vi "SafeBounds.vi"(5 "System no.":i32=1 min=1 step=1, 6 "Position":dbl[](array[numeric]), 7 "Type of movement":enum16{"Relative -", "Relative +", "Absolute"}(ring), 8 "Axes to move":string[](array[string]), 9 "Move":dbl[](array[numeric]), 10 "SafeMax":dbl[](array[numeric]) format="%.6f", 11 "SafeMin":dbl[](array[numeric]) format="%.6f") -> (1 "Faulty Axes":string, 2 "Message":string, 3 "All good?":bool)   [LabVIEW 2013]
panel:
  out "Moveable Axes":string[](array[string])
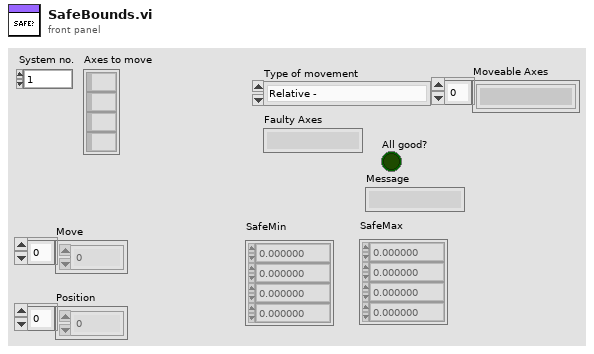
[diagram p1: front panel]
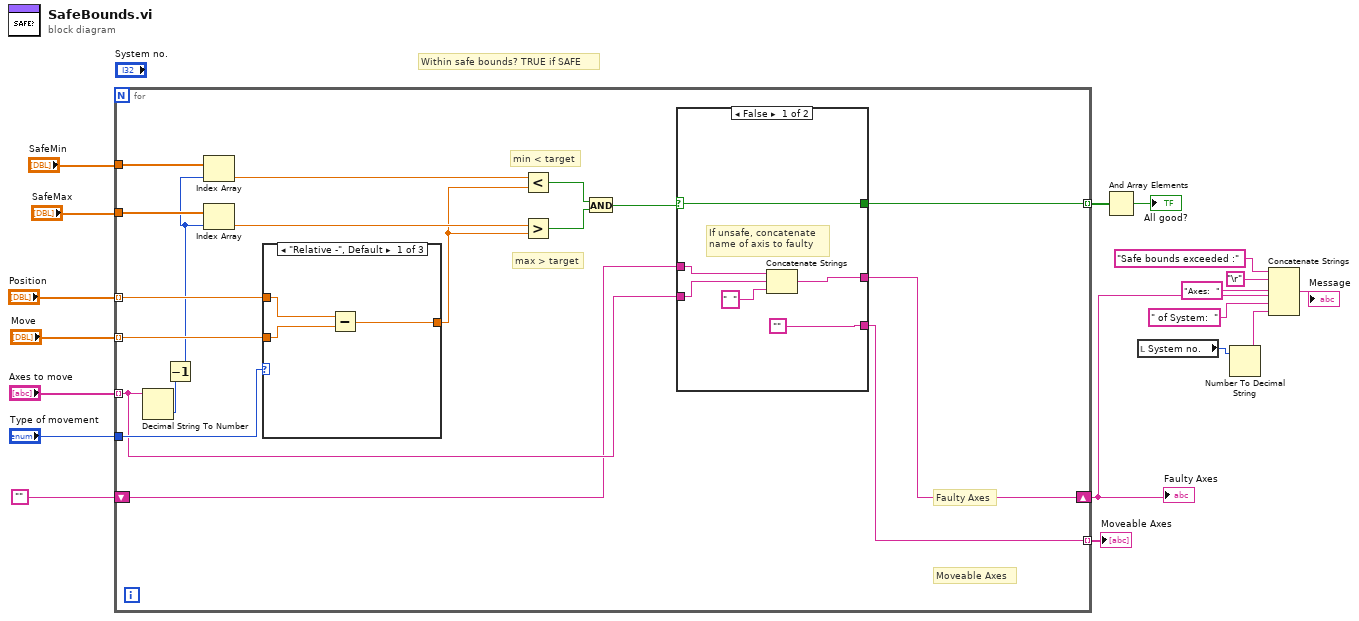
[diagram p0: block diagram]
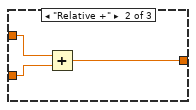
[diagram p3: hidden frame]
diagram:
  # "Within safe bounds? TRUE if SAFE"
  n1 = for {
    tunnel: "Axes to move" -> [w26] mode=indexing
    tunnel: "Position" -> [w21] mode=indexing
    tunnel: "Move" -> [w22] mode=indexing
    tunnel: "SafeMin" -> [w36]
    tunnel: "SafeMax" -> [w35]
    tunnel: "Type of movement" -> [w28]
    shift-right: [w24] -> w8
    shift-left: "" -> [w25]
    tunnel: [w23] -> w11 mode=indexing
    tunnel: [w19] -> w1 mode=indexing
    # "Moveable Axes"
    # "Faulty Axes"
    # "max > target"
    # "min < target"
    n2 = Decimal String To Number(string=w26) -> (number=w34:i32)  [unwired: 2 in, 1 out]
    n3 = Decrement(x=w34) -> (x-1=w20:i32)
    n4 = Index Array(array=w36, index=w20) -> (element=w32:dbl)
    n5 = Index Array(array=w35, index=w20) -> (element=w33:dbl)
    n6 = case shown="\"Relative -\", Default" w28 {
      tunnel: w21 -> [w48 w51 _]
      tunnel: [w47 w50 w52] -> w31
      tunnel: w22 -> [w46 w49 w52]
      frame "Relative -", Default {
        n7 = Subtract(x=w48, y=w46) -> (x-y=w47:dbl)
      }
      frame "Relative +" {
        n8 = Add(x=w51, y=w49) -> (x+y=w50:dbl)
      }
      frame "Absolute" {
      }
    }
    n9 = Less?(x=w32, y=w31) -> (x < y?=w30:bool)
    n10 = Greater?(x=w33, y=w31) -> (0:w29:bool)
    n11 = And(x=w30, y=w29) -> (x .and. y?=w27:bool)
    n12 = case shown="False" w27 {
      selector: w27 -> [w40 w44]
      tunnel: w26 -> [w38 w43]
      tunnel: w25 -> [w42 w45]
      tunnel: [w41 w45] -> w24
      tunnel: [w40 w44] -> w23
      tunnel: ["" w43] -> w19
      frame False {
        # "If unsafe, concatenate \nname of axis to faulty"
        n13 = Concatenate Strings(w42, w38, "  " ("string")) -> (w41:string)
      }
      frame True {
        # "If safe, don't concatenate \nname of axis to faulty"
      }
    }
  }
  "Faulty Axes" <- w8
  "Moveable Axes" <- w1
  n14 = And Array Elements(Boolean array=w11) -> (logical AND=→"All good?":bool)
  n15 = local read "System no."() -> (w6:i32)
  n16 = Number To Decimal String(number=w6) -> (decimal integer string=w5:string)  [unwired: 1 in]
  n17 = Concatenate Strings("Safe bounds exceeded :" ("message"), "\r", "Axes:  ", w8, " of System:  ", w5) -> (→"Message":string)
